vi "NTV_Drive On OFF.vi"(7 "Read(f) Write(t)":bool, 11 "Run Stop":bool=TRUE) -> (3 "Run Stop Out":bool=TRUE)   [LabVIEW 2023]
uses:
  <vilib>/Rock Robotics/Network Tables/NT Read Boolean.vi
  <vilib>/Rock Robotics/Network Tables/NT Write Boolean.vi
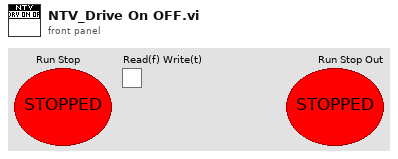
[diagram p1: front panel]
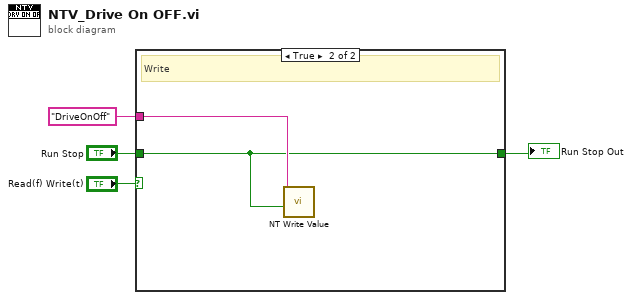
[diagram p0: block diagram]
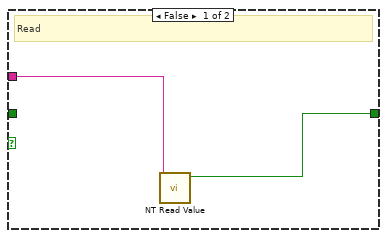
[diagram p2: hidden frame]
diagram:
  n1 = case shown="True" "Read(f) Write(t)" {
    tunnel: "Run Stop" -> [_ w7]
    tunnel: "DriveOnOff" ("Name") -> [w6 w8]
    tunnel: [w5 w7] -> w1
    frame False {
      # "Read"
      n2 = call-poly <vilib>:"NT Read Value.vi"("name"=w6) -> ("value"=w5:bool)  [unwired: 8 in, 2 out]
    }
    frame True {
      # "Write"
      n3 = call-poly <vilib>:"NT Write Value.vi"("value"=w7, "name"=w8) -> ()  [unwired: 9 in, 1 out]
    }
  }
  "Run Stop Out" <- w1
